vi "Useless Machine multithread test.vi"   [LabVIEW 2014]
uses:
  <vilib>/NXT/Block Support/NXT_InputPort.ctl
  <vilib>/NXT/Block Support/NXT_OutputPort.ctl
  <vilib>/NXT/Dual Mode Library/Waits/Wait_LetGo.vi
  <vilib>/NXT/Dual Mode Library/Waits/Wait_Touch.vi
  <vilib>/NXT/NXTIO Xnodes/NXTIONodeSubVIs/NXTMoveMotors.vi
  <vilib>/NXT/NXTIO Xnodes/NXTIONodeSubVIs/NXTStopMotors.vi
  <vilib>/NXT/NXTIO Xnodes/AddressXNode/NXTIOAddress.xnode
  <vilib>/NXT/NXTIO Xnodes/NXTIOXNode/NXTIO.xnode
  <vilib>/NXT/Subs/LVHSConnector.ctl
  <vilib>/NXT/LegoClasses/BrickReference/BrickReference.lvclass
types:
  T1 = typedef "NXT_InputPort.ctl" = u32
  T2 = typedef "NXT_OutputPort.ctl" = u8
  T3 = typedef "LVHSConnector.ctl" = refnum<class "BrickReference.lvclass">
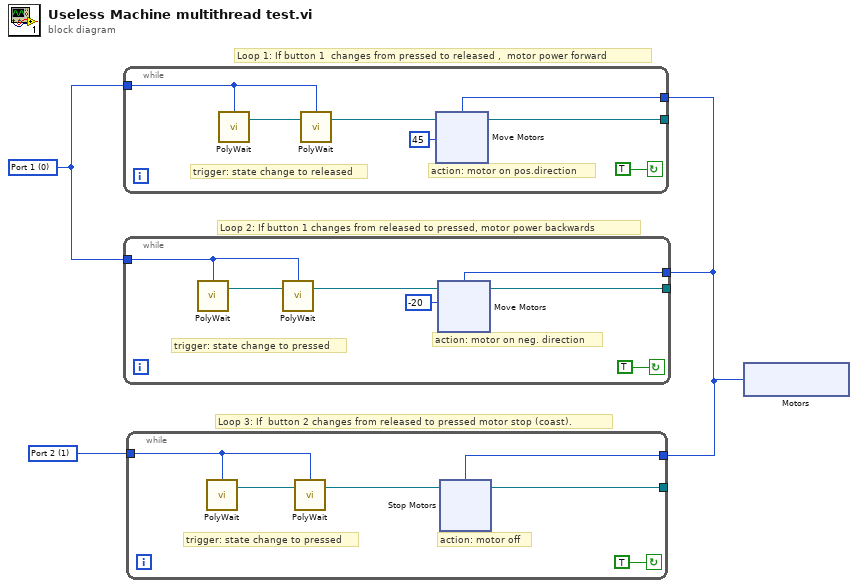
[diagram p0: block diagram]
diagram:
  w2 = T1 1 items=["Port 1", "Port 2", "Port 3", "Port 4"] ("Port (Port 1)")
  w3 = T1 0 items=["Port 1", "Port 2", "Port 3", "Port 4"] ("Port (Port 1)")
  # "Loop 3: If  button 2 changes from released to pressed motor stop (coast)."
  # "Loop 2: If button 1 changes from released to pressed, motor power backwards"
  # "Loop 1: If button 1  changes from pressed to released ,  motor power forward"
  n1 = xnode "Motors"() -> ("Motor"=w1:T2)
  n2 = while {
    tunnel: [w9] -> _
    tunnel: w3 -> [w5]
    tunnel: w1 -> [w4]
    stop <- TRUE continue-if-true
    # "action: motor on pos.direction"
    # "trigger: state change to released"
    n3 = call-poly <vilib>:"PolyWait.vi"("Port (Port 1)"=w5) -> ("NXT/EV3"=w6:T3)  [unwired: 3 in]
    n4 = call-poly <vilib>:"PolyWait.vi"("NXT/EV3"=w6, "Port (Port 1)"=w5) -> ("NXTEV3"=w10:T3)  [unwired: 2 in]
    n5 = xnode "Move Motors"("Power/Speed 1"=i8 45, "Motors"=w4, "NXT/EV3"=w10) -> ("NXT/EV3"=w9:T3)
  }
  n6 = while {
    tunnel: [w22] -> _
    tunnel: w3 -> [w19]
    tunnel: w1 -> [w18]
    stop <- TRUE continue-if-true
    # "action: motor on neg. direction"
    # "trigger: state change to pressed"
    n7 = call-poly <vilib>:"PolyWait.vi"("Port (Port 1)"=w19) -> ("NXTEV3"=w20:T3)  [unwired: 3 in]
    n8 = call-poly <vilib>:"PolyWait.vi"("NXT/EV3"=w20, "Port (Port 1)"=w19) -> ("NXT/EV3"=w23:T3)  [unwired: 2 in]
    n9 = xnode "Move Motors"("Power/Speed 1"=i8 -20, "Motors"=w18, "NXT/EV3"=w23) -> ("NXT/EV3"=w22:T3)
  }
  n10 = while {
    tunnel: [w37] -> _
    tunnel: w2 -> [w32]
    tunnel: w1 -> [w34]
    stop <- TRUE continue-if-true
    # "action: motor off"
    # "trigger: state change to pressed"
    n11 = call-poly <vilib>:"PolyWait.vi"("Port (Port 1)"=w32) -> ("NXTEV3"=w33:T3)  [unwired: 3 in]
    n12 = call-poly <vilib>:"PolyWait.vi"("NXT/EV3"=w33, "Port (Port 1)"=w32) -> ("NXT/EV3"=w35:T3)  [unwired: 2 in]
    n13 = xnode "Stop Motors"("Motors"=w34, "NXT/EV3"=w35) -> ("NXT/EV3"=w37:T3)
  }
